vi "Recursive Find Items.vi"(7 "$Path or Item Name":string, 8 "error in (no error)":errorcluster, 11 "JSON Schema in":string) -> (0 "error out":errorcluster, 1 "<JSON> Items":string[](array[string]) caption="<JSON>Items", 3 "Item Names":string[](array[string]), 4 "JSON Value Types":T1[](array[typedef]))   [LabVIEW 2019, in "JSON-Schema.lvlib"]
uses:
  JSON-Schema.lvlib
  <vilib>/JDP Science/JSONtext/JSON Value Type.ctl
  <vilib>/JDP Science/JSONtext/String Subset.vi
  <vilib>/JDP Science/JSONtext/support/Strip Quotes and Unescape.vi
  <vilib>/JDP Science/JSONtext/support/Unescape JSON string.vi
  <vilib>/JDP Science/JSONtext/Parsing/Parse Full Path or Item Name.vi
  <vilib>/JDP Science/JSONtext/Offset/Find Item Locations by Path.vi
  <vilib>/JDP Science/JSONtext/JSONtext.lvlib
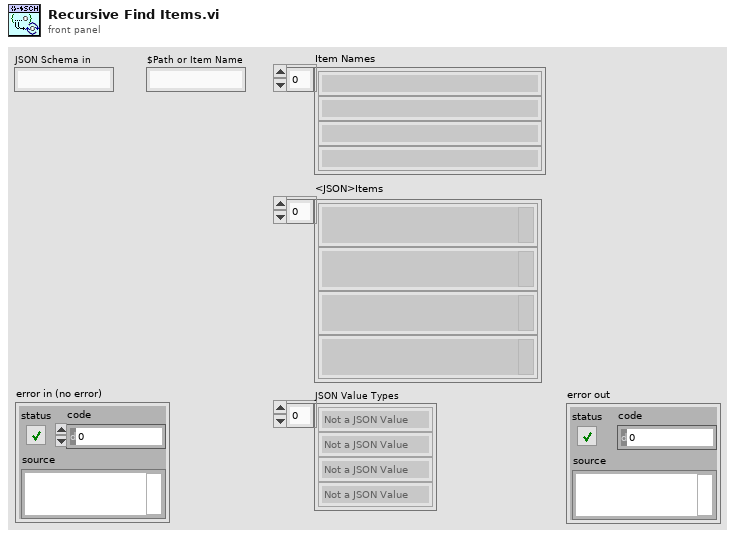
[diagram p1: front panel]
types:
  T1 = typedef "JSONtext.lvlib/JSON Value Type.ctl" = enum16{"Not a JSON Value", "JSON Object", "JSON Array", "String", "Number", "true", "false", "null"}
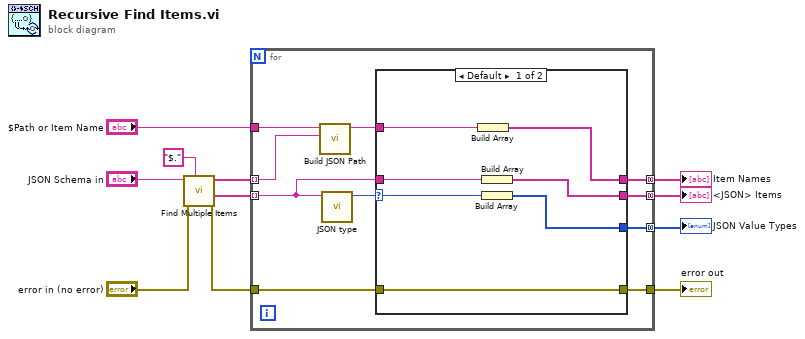
[diagram p0: block diagram]
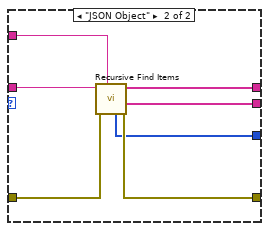
[diagram p2: hidden frame]
diagram:
  n1 = call <vilib>:"Find Multiple Items.vi"("$Path or Item Name"="$." ("string/path"), "error in (no error)"="error in (no error)", "JSON"="JSON Schema in") -> ("error out"=w8:errorcluster, "<JSON>"=w11:string[], "Item Names"=w6:string[])  [unwired: 5 in, 1 out]
  n2 = for {
    tunnel: w11 -> [w16] mode=indexing
    tunnel: w8 -> [w21]
    tunnel: [w20] -> w7
    tunnel: w6 -> [w12] mode=indexing
    tunnel: [w19] -> w5 mode=concatenating
    tunnel: [w18] -> w4 mode=concatenating
    tunnel: "$Path or Item Name" -> [w14]
    tunnel: [w15] -> w2 mode=concatenating
    n3 = call "Build JSON Path.vi"("Child element"=w12, "Base $Path"=w14) -> ("$Path out"=w13:string)  [unwired: 9 in]
    n4 = call <vilib>:"JSON type.vi"("JSON"=w16) -> ("JSON Value Type"=w17:T1)  [unwired: 9 in, 1 out]
    n5 = case shown="Default" w17 {
      selector: w17 -> [w25 _]
      tunnel: w21 -> [w27 w35]
      tunnel: [w27 w34] -> w20
      tunnel: w16 -> [w28 w33]
      tunnel: [w26 w31] -> w19
      tunnel: [w23 w32] -> w18
      tunnel: [w24 w30] -> w15
      tunnel: w13 -> [w22 w29]
      frame Default {
        n6 = Build Array(w22) -> (w26:string[])
        n7 = Build Array(w28) -> (w23:string[])
        n8 = Build Array(w25) -> (w24:T1[])
      }
      frame "JSON Object" {
        n9 = call "Recursive Find Items.vi"("$Path or Item Name"=w29, "error in (no error)"=w35, "JSON Schema in"=w33) -> ("error out"=w34:errorcluster, "<JSON> Items"=w32:string[], "Item Names"=w31:string[], "JSON Value Types"=w30:T1[])  [unwired: 5 in]
      }
    }
  }
  "error out" <- w7
  "Item Names" <- w5
  "<JSON> Items" <- w4
  "JSON Value Types" <- w2
